vi "Precess_coords_test.vi"() -> ()   [LabVIEW 2010]
panel:
  in  "Eq3":dbl=2012.159
  in  "Eq2":dbl=2012.159
  in  "Eq1":dbl=2000.0
  out "DEC (SN)":dbl format="%<%H:%M:%S%3u>t"
  out "RA (SN)":dbl format="%<%H:%M:%S%3u>t"
  out "DEC 2":dbl format="%<%H:%M:%S%3u>t"
  out "RA 2":dbl format="%<%H:%M:%S%3u>t"
  in  "DEC 2":dbl format="%<%H:%M:%S%3u>t"
  in  "RA 1":dbl format="%<%H:%M:%S%3u>t"
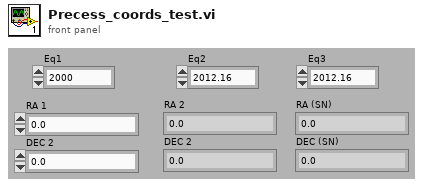
[diagram p1: front panel]
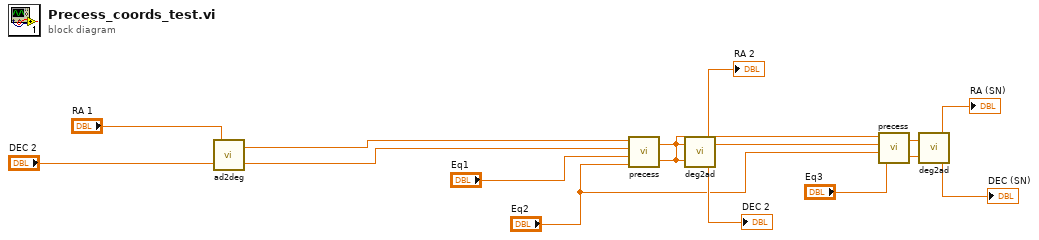
[diagram p0: block diagram]
diagram:
  n1 = call "ad2deg.vi"("DEC (sec)"="DEC 2", "RA (sec)"="RA 1") -> ("DEC (°)"=w11:dbl, "RA (°)"=w12:dbl)
  n2 = call "precess.vi"("Eq2"="Eq2", "Eq1"="Eq1", "DEC 1"=w11, "RA 1"=w12) -> ("DEC 2"=w8:dbl, "RA 2"=w9:dbl)
  n3 = call "deg2ad.vi"("DEC (°)"=w8, "RA (°)"=w9) -> ("DEC (sec)"=→"DEC 2":dbl, "RA (sec)"=→"RA 2":dbl)
  n4 = call "precess.vi"("Eq2"="Eq3", "Eq1"="Eq2", "DEC 1"=w8, "RA 1"=w9) -> ("DEC 2"=w4:dbl, "RA 2"=w5:dbl)
  n5 = call "deg2ad.vi"("DEC (°)"=w4, "RA (°)"=w5) -> ("DEC (sec)"=→"DEC (SN)":dbl, "RA (sec)"=→"RA (SN)":dbl)
